vi "StringToByteArray.vi"(6 "count":u32=1, 7 "isBigEndian":bool=TRUE, 8 "error in":errorcluster {"code" format="%.0x"}, 9 "numBytes":u32=1, 10 "Before":string, 11 "ResponseStringIn (01 23 45 67 89 AB CD EF FF EE)":string="01 23 45 67 89 AB CD EF FF EE") -> (0 "errorout":errorcluster {"code" format="%.0x"}, 1 "Array":u8[](array[numeric]) format="%.0x", 3 "ResponseStringOut":string)   [LabVIEW 2011, in "Agilent 546XX Series.lvlib"]
uses:
  Agilent 546XX Series.lvlib
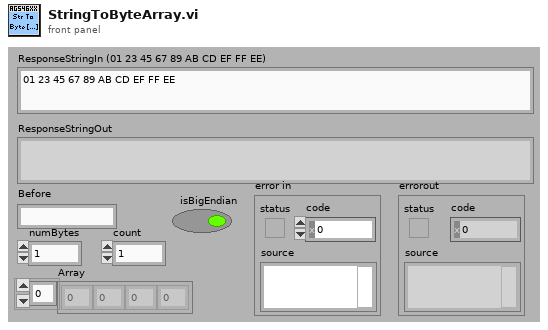
[diagram p1: front panel]
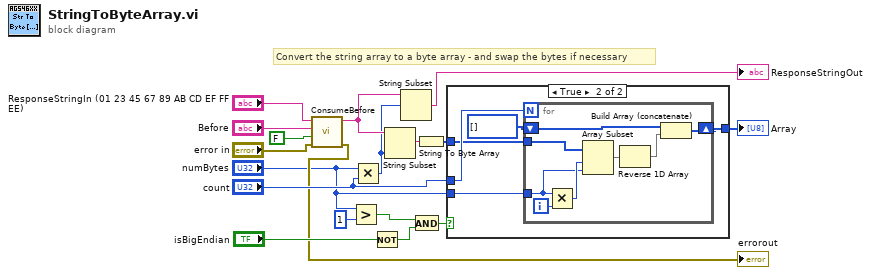
[diagram p0: block diagram]
diagram:
  # "Convert the string array to a byte array - and swap the bytes if necessary"
  n1 = call "ConsumeBefore.vi"("error in"="error in", "ASCII"=FALSE, "Before"="Before", "Response String In"="ResponseStringIn (01 23 45 67 89 AB CD EF FF EE)") -> ("error out"=→"errorout":errorcluster, "Response String Out"=w12:string)  [unwired: 6 in]
  n2 = Greater?(x="numBytes", y=u32 1) -> (0:w7:bool)
  n3 = Multiply(x="numBytes", y="count") -> (x*y=w10:u32)
  n4 = Not(x="isBigEndian") -> (.not. x?=w2:bool)
  n5 = String Subset(string=w12, length (rest)=w10) -> (substring=w13:string)  [unwired: 1 in]
  n6 = String Subset(string=w12, offset (0)=w10) -> (substring=→"ResponseStringOut":string)  [unwired: 1 in]
  n7 = And(x=w7, y=w2) -> (x .and. y?=w9:bool)
  n8 = String To Byte Array(string=w13) -> (unsigned byte array=w14:u8[])
  n9 = case shown="True" w9 {
    tunnel: w14 -> [w19 w23]
    tunnel: [w19 w21] -> w17
    tunnel: "count" -> [_ w24]
    tunnel: "numBytes" -> [_ w22]
    frame False {
    }
    frame True {
      n10 = for {
        N: w24 -> [_]
        tunnel: w23 -> [w32]
        tunnel: w22 -> [w29]
        shift-right: [w26] -> w21
        shift-left: u8[] [] -> [w25]
        i -> [w31]
        n11 = Multiply(x=w29, y=w31) -> (x*y=w30:u32)
        n12 = Array Subset(array=w32, index=w30, length=w29) -> (w28:u8[])
        n13 = Reverse 1D Array(array=w28) -> (reversed array=w27:u8[])
        n14 = Build Array (concatenate)(w25, w27) -> (w26:u8[])
      }
    }
  }
  "Array" <- w17
